vi "getDataTypeFromStrCntnt.vi"(8 "error in (no error)":errorcluster, 10 "strCntnt":string, 11 "Topic in":refnum<class "Topic.lvclass">) -> (0 "error out":errorcluster, 1 "strCntntLeft":string, 2 "dataType":string, 3 "Topic out":refnum<class "Topic.lvclass">)   [LabVIEW 2018, in "Topic.lvclass"]
doc: "Get the data type from string content."
uses:
  Topic.lvclass
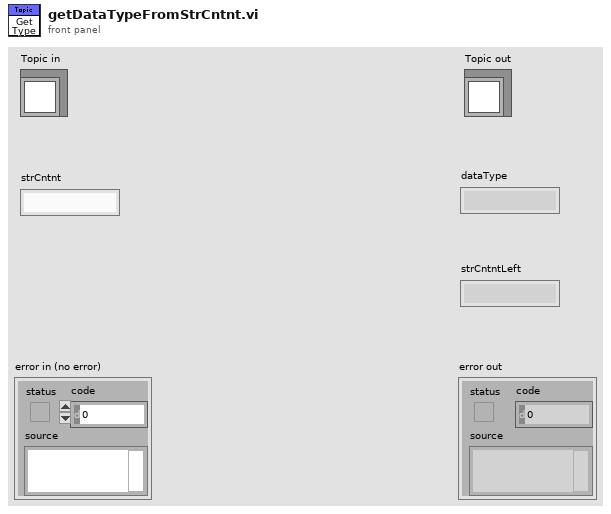
[diagram p1: front panel]
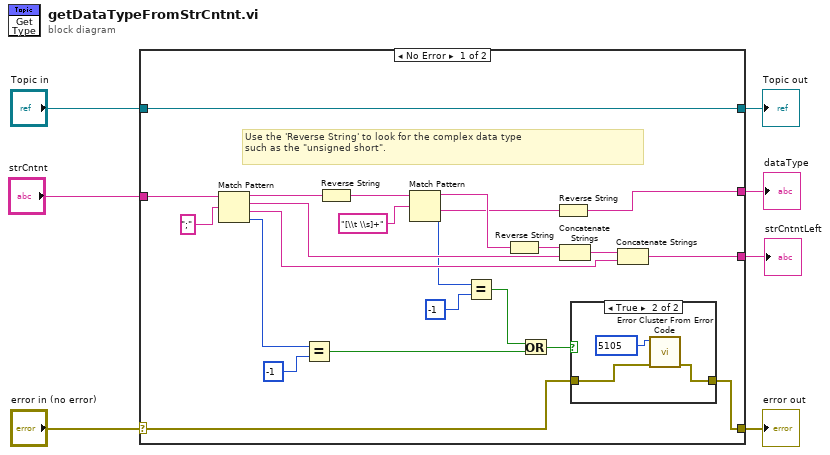
[diagram p0: block diagram]
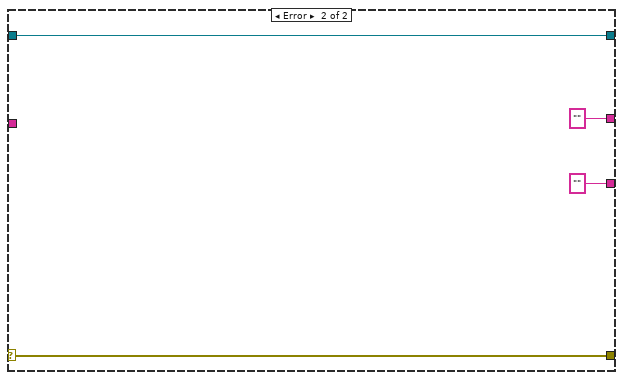
[diagram p3: hidden frame]
diagram:
  n1 = case shown="No Error" "error in (no error)" {
    selector: "error in (no error)" -> [w9 w38]
    tunnel: [w8 w38] -> w6
    tunnel: [w30 w37] -> w4
    tunnel: "Topic in" -> [w30 w37]
    tunnel: "strCntnt" -> [w19 _]
    tunnel: [w18 ""] -> w2
    tunnel: [w17 ""] -> w1
    frame No Error {
      # "Use the 'Reverse String' to look for the complex data type\nsuch as the \"unsigned short\"."
      n2 = Match Pattern(string=w19, regular expression=";") -> (before substring=w23:string, match substring=w27:string, after substring=w29:string, offset past match=w15:i32)  [unwired: 1 in]
      n3 = Equal?(x=w15, y=-1) -> (x = y?=w11:bool)
      n4 = Reverse String(1:w23) -> (0:w22:string)
      n5 = Match Pattern(string=w22, regular expression="[\\t \\s]+") -> (before substring=w25:string, after substring=w24:string, offset past match=w13:i32)  [unwired: 1 in, 1 out]
      n6 = Equal?(x=w13, y=-1) -> (x = y?=w12:bool)
      n7 = Reverse String(1:w25) -> (0:w26:string)
      n8 = Or(x=w12, y=w11) -> (x .or. y?=w10:bool)
      n9 = Reverse String(1:w24) -> (0:w17:string)
      n10 = Concatenate Strings(w26, w27) -> (w28:string)
      n11 = case shown="True" w10 {
        tunnel: w9 -> [w31 w33]
        tunnel: [w31 w32] -> w8
        frame False {
        }
        frame True {
          n12 = call <vilib>:"Error Cluster From Error Code.vi"("error in (no error)"=w33, "error code (0)"=5105) -> ("error out"=w32:errorcluster)  [unwired: 7 in]
        }
      }
      n13 = Concatenate Strings(w28, w29) -> (w18:string)
    }
    frame Error {
    }
  }
  "error out" <- w6
  "Topic out" <- w4
  "dataType" <- w1
  "strCntntLeft" <- w2
